vi "Handshake.vi"(8 "error in (no error)":errorcluster, 11 "Connection.TCP in":refnum<class "Connection.TCP.lvclass">) -> (0 "error out":errorcluster, 3 "Connection.TCP out":refnum<class "Connection.TCP.lvclass">)   [LabVIEW 2013]
uses:
  Connection.TCP.lvclass
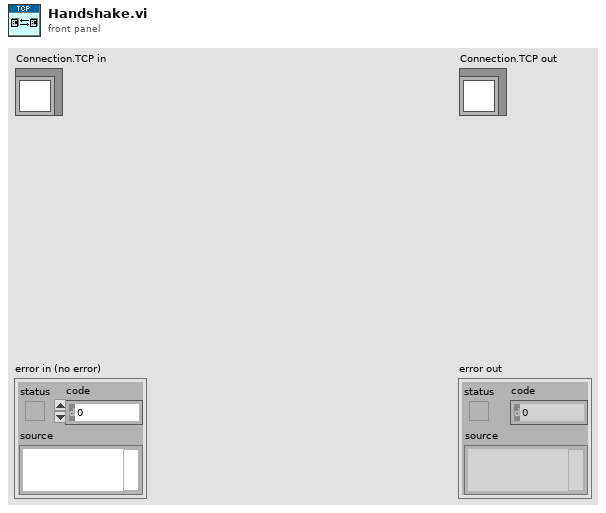
[diagram p1: front panel]
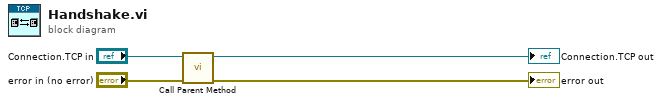
[diagram p0: block diagram]
diagram:
  n1 = call-parent "Call Parent Method"("error in (no error)"="error in (no error)", "Connection in"="Connection.TCP in") -> ("error out"=→"error out":errorcluster, "Connection out"=→"Connection.TCP out":refnum<class "Connection.TCP.lvclass">)  [unwired: 8 in]
